vi "_Write.vi"(8 "error in (no error)":errorcluster, 10 "Data":string, 11 "TCPStreamProxy in":refnum<class "TCPStream.lvclass">) -> (0 "error out":errorcluster, 3 "TCPStreamProxy out":refnum<class "TCPStream.lvclass">)   [LabVIEW 2020, in "HTTP Utils.lvlib" / "TCPStream.lvclass"]
uses:
  TCPStream.lvclass
  TCPStream.lvclass/TCPStream.ctl
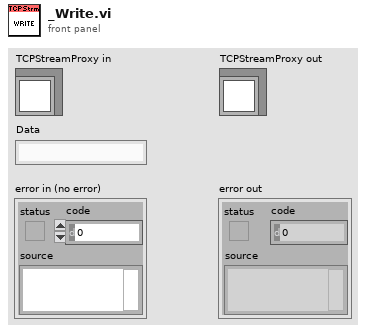
[diagram p1: front panel]
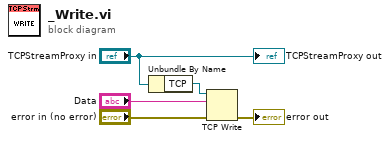
[diagram p0: block diagram]
diagram:
  n1 = Unbundle By Name("TCPStreamProxy in") -> ("TCP"=w4:refnum<k5>)
  n2 = TCP Write(connection ID=w4, data in="Data", error in (no error)="error in (no error)") -> (error out=→"error out":errorcluster)  [unwired: 1 in, 2 out]
  "TCPStreamProxy out" <- "TCPStreamProxy in"
